vi "TorqueCurrentFOC Setter.vi"(0 "DeviceReference":T1, 3 "Update Frequency (Hz)":dbl=100.0, 5 "Output":dbl, 7 "MaxAbsDutyCycle":dbl=1.0, 9 "Deadband":dbl) -> (4 "DeviceReference Out":T1)   [LabVIEW 2020]
doc: "Request a specified motor current (field oriented control).\nThis control request will drive the motor to the requested motor (stator) current value. This leverages field oriented control (FOC), which means greater peak power than what is documented. This scales to torque based on Motor's kT constant."
uses:
  DeviceReference.ctl
  <userlib>/CTRE_PhoenixTools/CTRE_PhoenixTools.lvlib
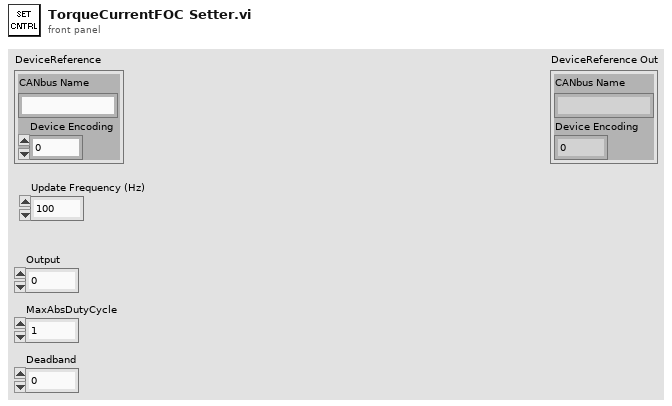
[diagram p1: front panel]
types:
  T1 = typedef "DeviceReference.ctl" = cluster{"CANbus Name":string, "Device Encoding":u32}
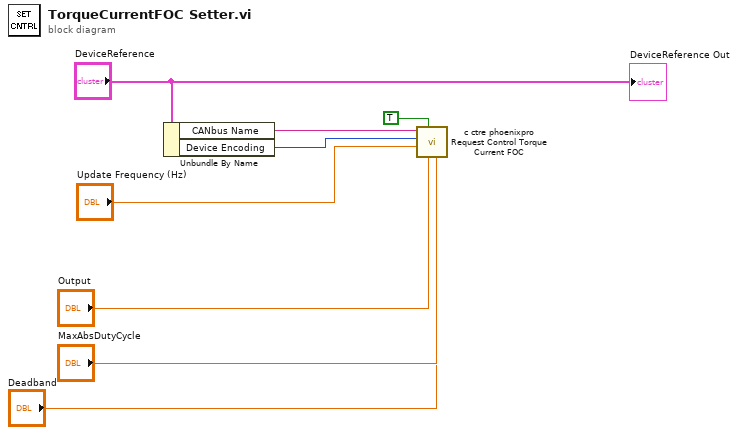
[diagram p0: block diagram]
diagram:
  n1 = Unbundle By Name("DeviceReference") -> ("CANbus Name"=w7:string, "Device Encoding"=w6:u32)
  n2 = call <userlib>:"c ctre phoenixpro Request Control Torque Current FOC.vi"("Deadband"="Deadband", "MaxAbsDutyCycle"="MaxAbsDutyCycle", "Output"="Output", "cancelOtherRequests"=TRUE, "updateTime"="Update Frequency (Hz)", "ecuEncoding"=w6, "canbus"=w7) -> ()  [unwired: 3 in, 2 out]
  "DeviceReference Out" <- "DeviceReference"
